vi "颗粒二值化.vi"() -> ()   [LabVIEW 2018]
uses:
  <vilib>/vision/NI_Vision_Development_Module.lvlib
panel:
  in  "停止":bool
  out "Region Reports":T1(array[cluster]) {"Mean Value" format="%.2f"; "%" format="%.2f"; "Area (calibrated)" format="%.2f"; "Maximal Value" format="%.2f"; "Minimal Value" format="%.2f"; "Standard Variation" format="%.2f"}
  out "Number of Particles":i32
  out "Image 2":T2(plugin-control)
  in  "Range":cluster{"Lower value":sgl, "Upper value":sgl} {"Upper value" format="%.2f"; "Lower value" format="%.2f"}
  out "Image":T2(plugin-control)
  in  "路径":path
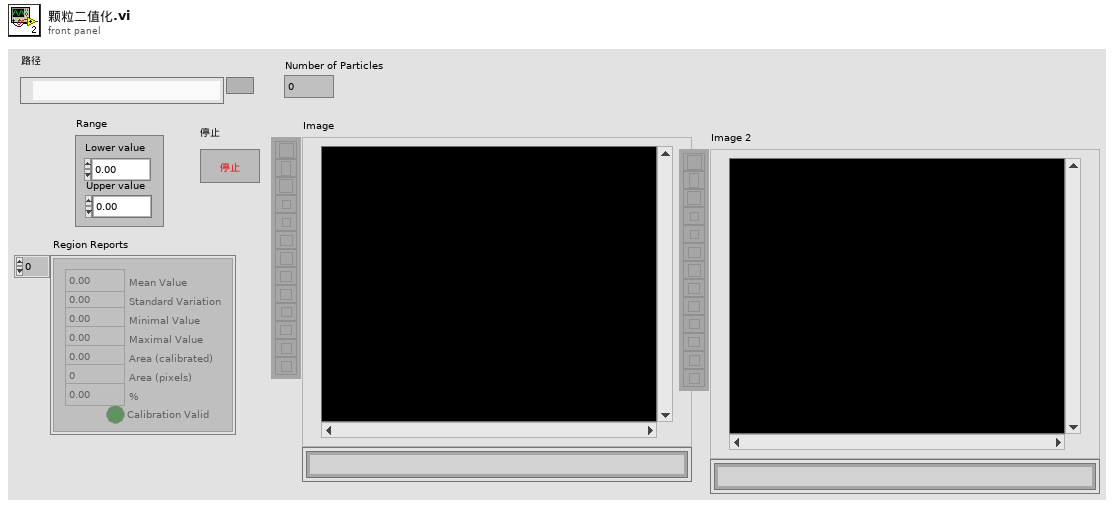
[diagram p1: front panel]
types:
  T1 = cluster{"Mean Value":sgl, "Standard Variation":sgl, "Minimal Value":sgl, "Maximal Value":sgl, "Area (calibrated)":sgl, "Area (pixels)":u32, "%":sgl, "Calibration Valid":bool}[]
  T2 = typedef "IMAQ Image.ctl" = refnum<image>
  T3 = enum32{"AutoM", "Close", "Dilate", "Erode", "Gradient", "Gradient out", "Gradient in", "Hit miss", "Open", "PClose", "POpen", "Thick", "Thin"}
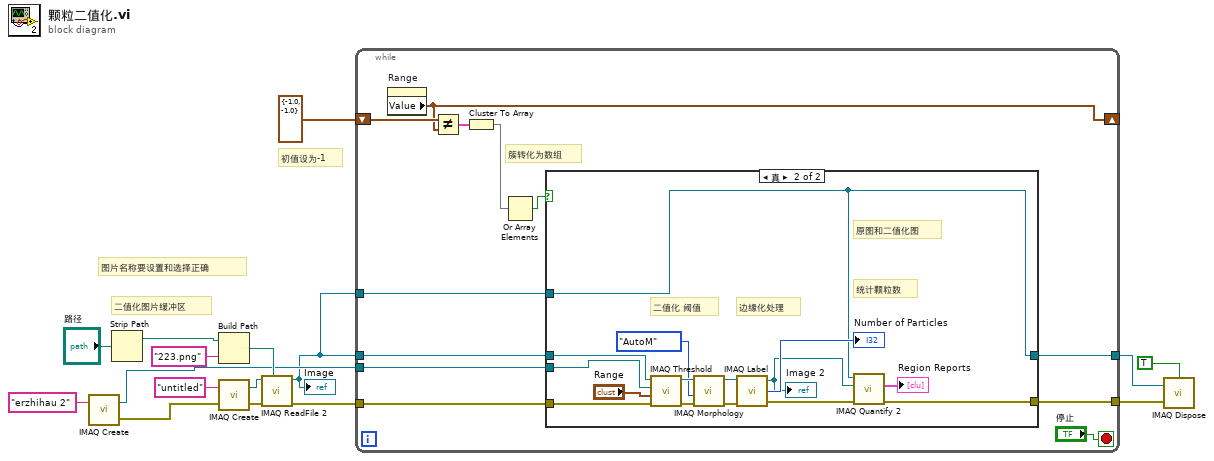
[diagram p0: block diagram]
diagram:
  # "图片名称要设置和选择正确"
  # "初值设为-1"
  # "二值化图片缓冲区"
  n1 = call "IMAQ Create"("Image Name"="erzhihau 2") -> ("New Image"=w7:T2, "error out"=w8:errorcluster)  [unwired: 4 in]
  n2 = Strip Path(path="路径") -> (stripped path=w16:path)  [unwired: 1 out]
  n3 = Build Path(base path=w16, name or relative path="223.png" ("名称或相对路径")) -> (appended path=w11:path)
  n4 = call "IMAQ Create"("Image Name"="untitled", "error in (no error)"=w8) -> ("New Image"=w12:T2, "error out"=w10:errorcluster)  [unwired: 3 in]
  n5 = call "IMAQ ReadFile 2"("File Path"=w11, "error in (no error)"=w10, "Image"=w12) -> ("error out"=w6:errorcluster, "Image Out"=w1:T2)  [unwired: 4 in, 3 out]
  "Image" <- w1
  n6 = while {
    tunnel: w7 -> [w28]
    tunnel: w1 -> [w27]
    tunnel: w6 -> [w26]
    shift-right: [w23] -> _
    shift-left: cluster{"Lower value":sgl, "Upper value":sgl} {"Lower value"=-1.0, "Upper value"=-1.0} ("x") -> [w25]
    tunnel: [w20] -> w4
    tunnel: [w19] -> w3
    tunnel: w1 -> [w17]
    stop <- "停止" stop-if-true
    # "簇转化为数组"
    n7 = property on="Range" class="Clust (严格)"() -> ("Value"=w23:cluster{"Lower value":sgl, "Upper value":sgl})  [unwired: 2 in, 2 out]
    n8 = Not Equal?(x=w25, y=w23) -> (x != y?=w24:cluster{"Lower value":bool, "Upper value":bool})
    n9 = Cluster To Array(cluster=w24) -> (array=w22:bool[])
    n10 = Or Array Elements(Boolean array=w22) -> (logical OR=w21:bool)
    n11 = case shown="真" w21 {
      tunnel: w28 -> [_ w45]
      tunnel: w27 -> [w30 w33]
      tunnel: w26 -> [w29 w44]
      tunnel: [w29 w35] -> w20
      tunnel: [w30 w31] -> w19
      tunnel: w17 -> [_ w31]
      frame False {
      }
      frame True {
        # "统计颗粒数"
        # "原图和二值化图"
        # "边缘化处理"
        # "二值化 阈值"
        n12 = call "IMAQ Threshold"("error in (no error)"=w44, "Range"="Range", "Image Dst"=w45, "Image Src"=w33) -> ("error out"=w41:errorcluster, "Image Dst Out"=w42:T2)  [unwired: 6 in]
        n13 = call "IMAQ Morphology"("error in (no error)"=w41, "Operation"=T3."AutoM", "Image Src"=w42) -> ("error out"=w40:errorcluster, "Image Dst Out"=w37:T2)  [unwired: 7 in]
        n14 = call "IMAQ Label"("error in (no error)"=w40, "Image Src"=w37) -> ("error out"=w36:errorcluster, "Number of Particles"=→"Number of Particles":i32, "Image Dst Out"=w38:T2)  [unwired: 2 in]
        "Image 2" <- w38
        n15 = call "IMAQ Quantify 2"("error in (no error)"=w36, "Image Mask"=w38, "Image"=w31) -> ("error out"=w35:errorcluster, "Region Reports"=→"Region Reports":T1)  [unwired: 6 in, 1 out]
      }
    }
  }
  n16 = call "IMAQ Dispose"("All Images? (No)"=TRUE, "Image"=w3, "error in (no error)"=w4) -> ()  [unwired: 3 in, 1 out]
